vi "Increment Version.vi"(6 "Revision Type String":string, 8 "error in (no error)":errorcluster, 10 "Previous Version":cluster{i32, i32, i32, i32}) -> (0 "error out":errorcluster, 2 "New Version":cluster{i32, i32, i32, i32})   [LabVIEW 2019]
doc: "Increments the Version Number according to the <b>Revision Type String</b>, which should be chosen from {MAJOR,MINOR,PATCH,BUILD}."
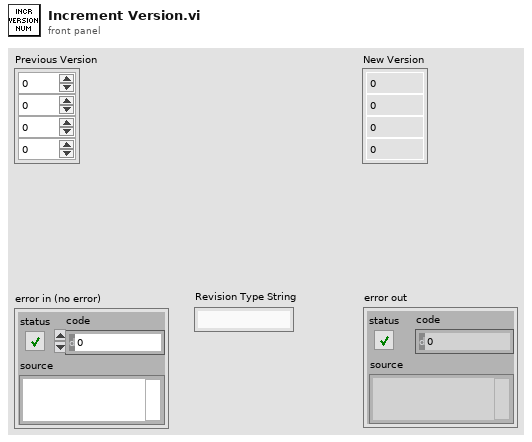
[diagram p1: front panel]
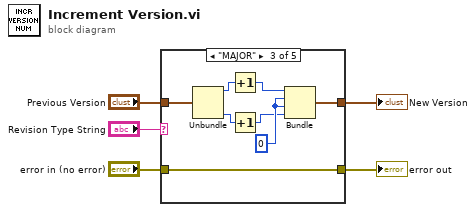
[diagram p0: block diagram]
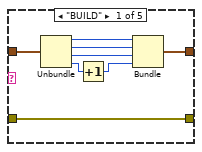
[diagram p2: hidden frame]
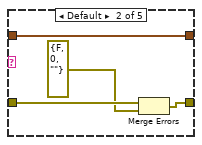
[diagram p3: hidden frame]
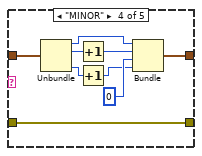
[diagram p4: hidden frame]
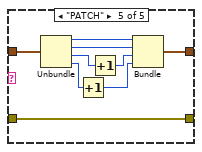
[diagram p5: hidden frame]
diagram:
  n1 = case shown="\"MAJOR\"" "Revision Type String" {
    tunnel: "Previous Version" -> [w13 w14 w20 w30 w40]
    tunnel: [w12 w14 w19 w29 w39] -> w3
    tunnel: "error in (no error)" -> [w6 w17 w24 w33 w43]
    tunnel: [w6 w16 w24 w33 w43] -> w1
    frame "BUILD" {
      n2 = Unbundle(w13) -> (w11:i32, w10:i32, w9:i32, w8:i32)
      n3 = Increment(x=w8) -> (x+1=w7:i32)
      n4 = Bundle(w11, w10, w9, w7) -> (w12:cluster{i32, i32, i32, i32})  [unwired: 1 in]
    }
    frame Default {
      n5 = Merge Errors(w17, errorcluster {"status"=FALSE, "code"=0, "source"=""} ("error constant")) -> (w16:errorcluster)
    }
    frame "MAJOR" {
      w25 = 0
      n6 = Unbundle(w20) -> (w23:i32, w22:i32)  [unwired: 2 out]
      n7 = Increment(x=w23) -> (x+1=w18:i32)
      n8 = Increment(x=w22) -> (x+1=w21:i32)
      n9 = Bundle(w18, w25, w25, w21) -> (w19:cluster{i32, i32, i32, i32})  [unwired: 1 in]
    }
    frame "MINOR" {
      n10 = Unbundle(w30) -> (w26:i32, w27:i32, w32:i32)  [unwired: 1 out]
      n11 = Increment(x=w27) -> (x+1=w28:i32)
      n12 = Increment(x=w32) -> (x+1=w31:i32)
      n13 = Bundle(w26, w28, 0, w31) -> (w29:cluster{i32, i32, i32, i32})  [unwired: 1 in]
    }
    frame "PATCH" {
      n14 = Unbundle(w40) -> (w38:i32, w35:i32, w37:i32, w42:i32)
      n15 = Increment(x=w42) -> (x+1=w41:i32)
      n16 = Increment(x=w37) -> (x+1=w36:i32)
      n17 = Bundle(w38, w35, w36, w41) -> (w39:cluster{i32, i32, i32, i32})  [unwired: 1 in]
    }
  }
  "New Version" <- w3
  "error out" <- w1
